vi "select single-cont.vi"(8 "error in":errorcluster, 9 "upper limit":bool, 10 "sprinkler data in":T1 {"Zone Indicators"."Timing" format="%#.2g"}, 11 "Controls":T6) -> (0 "error out":errorcluster, 2 "status":T5, 3 "sprinkler data out":T1 {"Zone Indicators"."Timing" format="%#.2g"})   [LabVIEW 2015]
uses:
  controls/state.ctl
  controls/sprinkler data.ctl
  Solution/Controls/Zone Setup.ctl
  Solution/Controls/Zone.ctl
  Solution/Controls/Zone Indicators.ctl
  controls/timer state.ctl
panel:
  # "Continuous"
  # "Single"
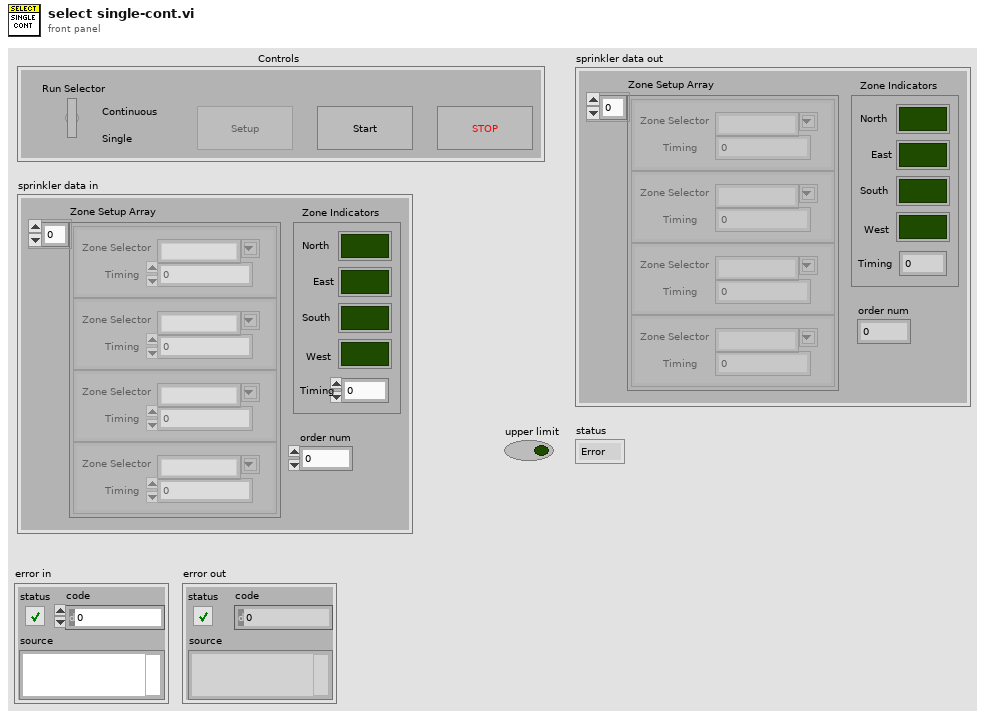
[diagram p1: front panel]
types:
  T1 = typedef "sprinkler data.ctl" = cluster{"Zone Setup Array":T2[], "Zone Indicators":T4, "order num":i32}
  T2 = typedef "Zone Setup.ctl" = cluster{"Zone Selector":T3, "Timing":u32}
  T3 = typedef "Zone.ctl" = string
  T4 = typedef "Zone Indicators.ctl" = cluster{"North":bool, "East":bool, "South":bool, "West":bool, "Timing":dbl}
  T5 = typedef "state.ctl" = enum16{"Error", "End", "Start", "Exit", "Setup", "Low pressure", "Rain", "Run", "Idle", "Initialize"}
  T6 = cluster{"Run Selector":bool, "Setup":bool, "Start":bool, "Stop":bool}
  T7 = typedef "timer state.ctl" = enum16{"Stop", "Start"}
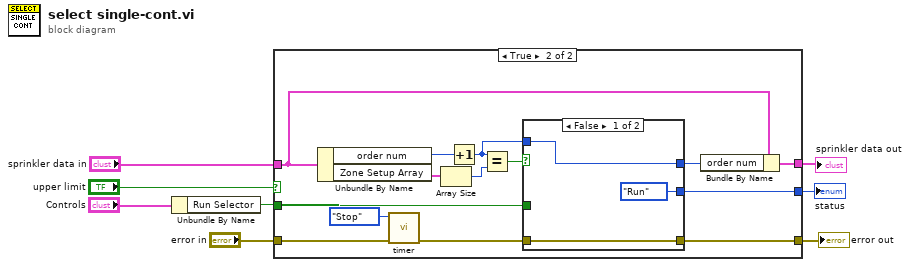
[diagram p0: block diagram]
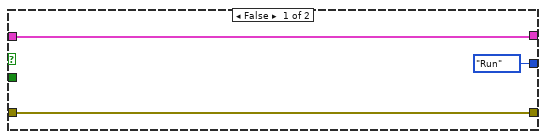
[diagram p2: hidden frame]
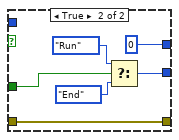
[diagram p3: hidden frame]
diagram:
  n1 = Unbundle By Name("Controls") -> ("Run Selector"=w6:bool)
  n2 = case shown="True" "upper limit" {
    tunnel: "sprinkler data in" -> [w11 w24]
    tunnel: w6 -> [_ w18]
    tunnel: [state."Run" ("status") w17] -> w7
    tunnel: [w11 w16] -> w8
    tunnel: "error in" -> [w9 w14]
    tunnel: [w9 w15] -> w1
    frame False {
    }
    frame True {
      n3 = Unbundle By Name(w24) -> ("order num"=w25:i32, "Zone Setup Array"=w22:T2[])
      n4 = call "timer.vi"("error in"=w14, "timer state"=timer_state."Stop") -> ("error out"=w13:errorcluster)  [unwired: 7 in, 2 out]
      n5 = Array Size(array=w22) -> (size(s)=w23:i32)
      n6 = Increment(x=w25) -> (x+1=w20:i32)
      n7 = Equal?(x=w20, y=w23) -> (x = y?=w21:bool)
      n8 = case shown="False" w21 {
        tunnel: w20 -> [w28 _]
        tunnel: [w28 0] -> w19
        tunnel: w18 -> [_ w34]
        tunnel: [state."Run" ("status") w30] -> w17
        tunnel: w13 -> [w26 w29]
        tunnel: [w26 w29] -> w15
        frame False {
        }
        frame True {
          n9 = Select(t=state."Run" ("status"), s=w34, f=state."End" ("status")) -> (s? t:f=w30:T5)
        }
      }
      n10 = Bundle By Name(cluster=w24, "order num"=w19) -> (w16:T1)
    }
  }
  "status" <- w7
  "sprinkler data out" <- w8
  "error out" <- w1
